vi "Write Y_limiter.vi"(8 "error in (no error)":errorcluster, 10 "Y_limiter":T1 {"output" format="%.2f"}, 11 "reg in":refnum<class "bronkhorst_reg_1.lvclass">) -> (0 "error out":errorcluster, 3 "reg out":refnum<class "bronkhorst_reg_1.lvclass">)   [LabVIEW 2019, in "bronkhorst_reg_1.lvclass"]
uses:
  bronkhorst_reg_1.lvclass
  ctl/Y_Lim_ext_defs.ctl
  ctl/Y_Lim_State.ctl
  bronkhorst_reg_1.lvclass/bronkhorst_reg_1.ctl
  control.lvlib
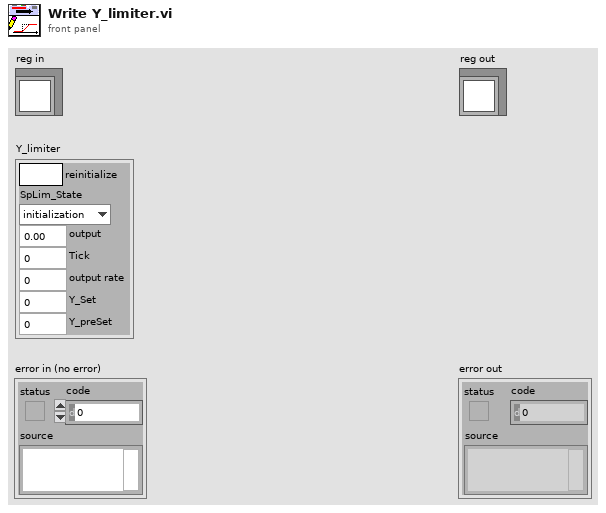
[diagram p1: front panel]
types:
  T1 = typedef "control.lvlib/Y_Lim_ext_defs.ctl" = cluster{"reinitialize":bool, "SpLim_State":T2, "output":dbl, "Tick":u32, "output rate":dbl, "Y_Set":dbl, "Y_preSet":dbl}
  T2 = typedef "control.lvlib/Y_Lim_State.ctl" = enum8{"initialization", "alarm", "stop", "decrease", "increase"}
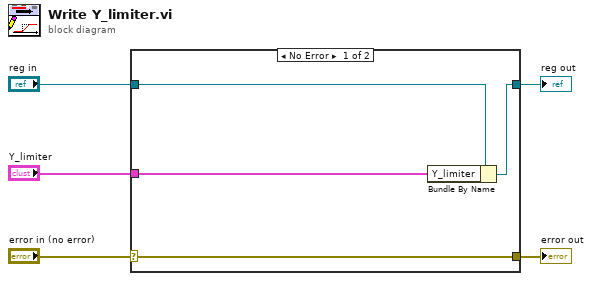
[diagram p0: block diagram]
diagram:
  n1 = case shown="No Error" "error in (no error)" {
    selector: "error in (no error)" -> [w9 w10]
    tunnel: [w9 w10] -> w4
    tunnel: [w7 w11] -> w2
    tunnel: "reg in" -> [w8 w11]
    tunnel: "Y_limiter" -> [w6 _]
    frame No Error {
      n2 = Bundle By Name(cluster=w8, "Y_limiter"=w6) -> (w7:refnum<class "bronkhorst_reg_1.lvclass">)
    }
    frame Error {
    }
  }
  "error out" <- w4
  "reg out" <- w2
